vi "enumerateStaticDependencies.vi"(8 "error in (no error)":errorcluster, 11 "SMO.DynamicLauncher":refnum<class "SMO.DynamicLauncher.lvclass">) -> (0 "error out":errorcluster, 2 "Static Dependencies":refnum<class "Dependency.lvclass">[](array[class]), 3 "SMO.DynamicLauncher out":refnum<class "SMO.DynamicLauncher.lvclass">)   [LabVIEW 2013, in "SMO.DynamicLauncher.lvclass"]
uses:
  SMO.DynamicLauncher.lvclass
  src/Dependency/Dependency.lvclass
  src/SMO/SMO.lvclass
panel:
  # "For instructions on how to use the JKI State Machine Objects, examples and video tutorials, visit:\nhttp://jki.net/state-machine-objects/\n\nJKI State Machine Objects™\nhttp://jki.net/state-machine-objects/\nCopyright (C) 2005-2015, JKI <info@jki.net>\nALL RIGHTS RESERVED"
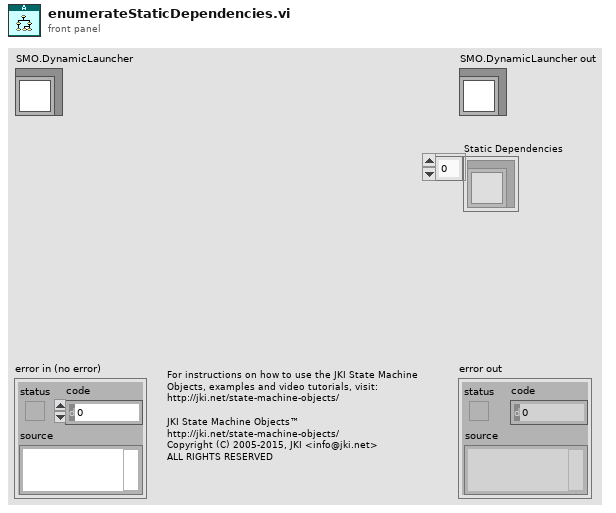
[diagram p1: front panel]
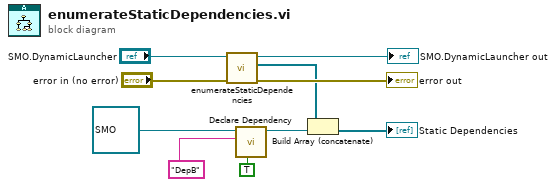
[diagram p0: block diagram]
diagram:
  n1 = call-parent "enumerateStaticDependencies.vi"("error in (no error)"="error in (no error)", "SMO"="SMO.DynamicLauncher") -> ("error out"=→"error out":errorcluster, "Static Dependencies"=w6:refnum<class "Dependency.lvclass">[], "SMO out"=→"SMO.DynamicLauncher out":refnum<class "SMO.DynamicLauncher.lvclass">)  [unwired: 7 in]
  n2 = call "Declare Dependency.vi"("Shared Resource (F)"=TRUE, "Name"="DepB", "Type"=refnum<class "SMO.lvclass"> refnum ("SMO.lvclass")) -> ("Dependency out"=w3:refnum<class "Dependency.lvclass">)  [unwired: 7 in, 1 out]
  n3 = Build Array (concatenate)(w6, w3) -> (→"Static Dependencies":refnum<class "Dependency.lvclass">[])
